vi "TestExec.Add Result Suffix to UUT Folder.vi"(10 "ResultState":T1, 11 "Path":path) -> (1 "Changed":bool, 3 "New Path":path)   [LabVIEW 2024]
uses:
  <vilib>/KATE/SeqMgr/SeqMgr.Result State Enum.ctl
  <vilib>/KATE/SeqMgr/SeqMgr.lvlib
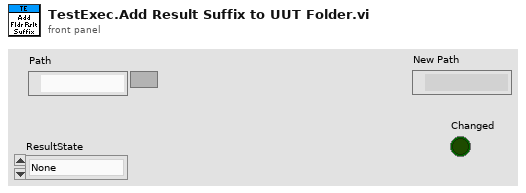
[diagram p1: front panel]
types:
  T1 = typedef "KATE_Lib.lvlib/SeqMgr.lvlib/SeqMgr.Result State Enum.ctl" = enum16{"None", "Passing", "Failing", "PASS", "FAIL", "ABORT", "ERROR"}
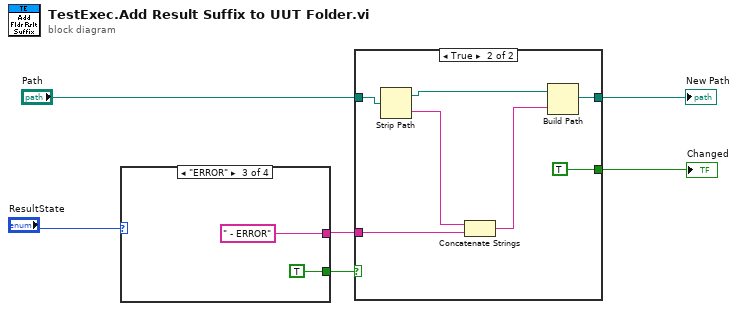
[diagram p0: block diagram]
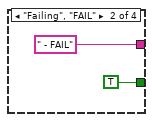
[diagram p4: hidden frame]
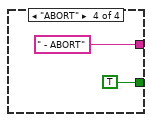
[diagram p5: hidden frame]
diagram:
  n1 = case shown="\"ERROR\"" "ResultState" {
    tunnel: [_ TRUE TRUE TRUE] -> w5
    tunnel: [_ " - FAIL" " - ERROR" " - ABORT"] -> w4
    frame "None", Default {
    }
    frame "Failing", "FAIL" {
    }
    frame "ERROR" {
    }
    frame "ABORT" {
    }
  }
  n2 = case shown="True" w5 {
    tunnel: w4 -> [_ w20]
    tunnel: "Path" -> [w13 w18]
    tunnel: [w13 w19] -> w2
    tunnel: [_ TRUE] -> w1
    frame False {
    }
    frame True {
      n3 = Strip Path(path=w18) -> (stripped path=w15:path, name=w17:string)
      n4 = Concatenate Strings(w17, w20) -> (w16:string)
      n5 = Build Path(base path=w15, name or relative path=w16) -> (appended path=w19:path)
    }
  }
  "New Path" <- w2
  "Changed" <- w1
